vi "Main.vi"() -> ()   [LabVIEW 2020]
uses:
  <vilib>/Utility/error.llb/DialogType.ctl
  TypeDefs/SN_Enum.ctl
  <vilib>/numeric/Random Number (Range) DBL.vi
  <vilib>/ErrorRing/Error Ring.xnode
  <vilib>/Utility/SystemLogging/NI_SystemLogging.lvlib
panel:
  out "notification 2":bool
  out "notification 4":bool
  out "notification 1":bool
  out "notification 3":bool
  in  "Start Button":bool
  in  "View Button":bool
  out "error out":errorcluster
  in  "Abort Button":bool
  out "Tab Control":enum32{"Page 0", "Page 1", "Page 2"}(tab)
  in  "Save Button":bool
  in  "Path Control":path
  out "Grafica de Control":dbl(graph) caption="Waveform Chart - Dark"
  out "Torque Read":dbl
  in  "Torque Write":dbl
  out "Torque Read 2":dbl
  in  "Torque Write 2":dbl
  out "Torque Read 3":dbl
  in  "Tabs Buttons":enum32{"Button 1", "Button 2", "Button 3"}(radio)
  out "First Call: T/F":bool
  # "Debbugging Additional Objects"
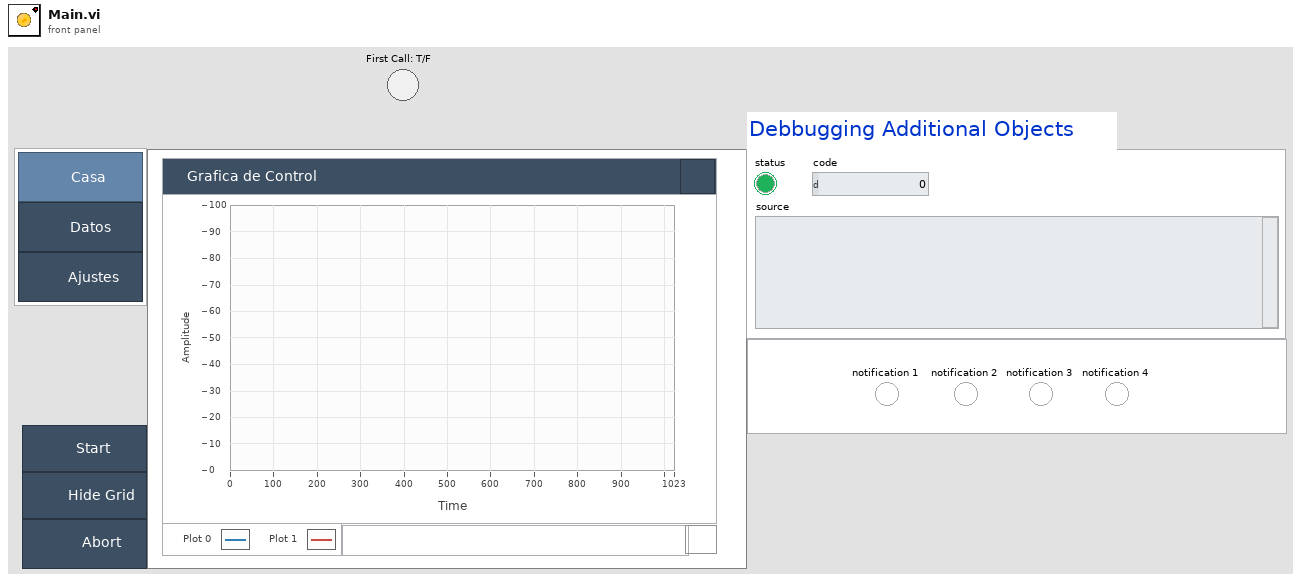
[diagram p1: front panel]
types:
  T1 = typedef "SN_Enum.ctl" = enum16{"Starting up", "Adquisition", "Save", "Fault"}
  T2 = typedef "DialogType.ctl" = u16
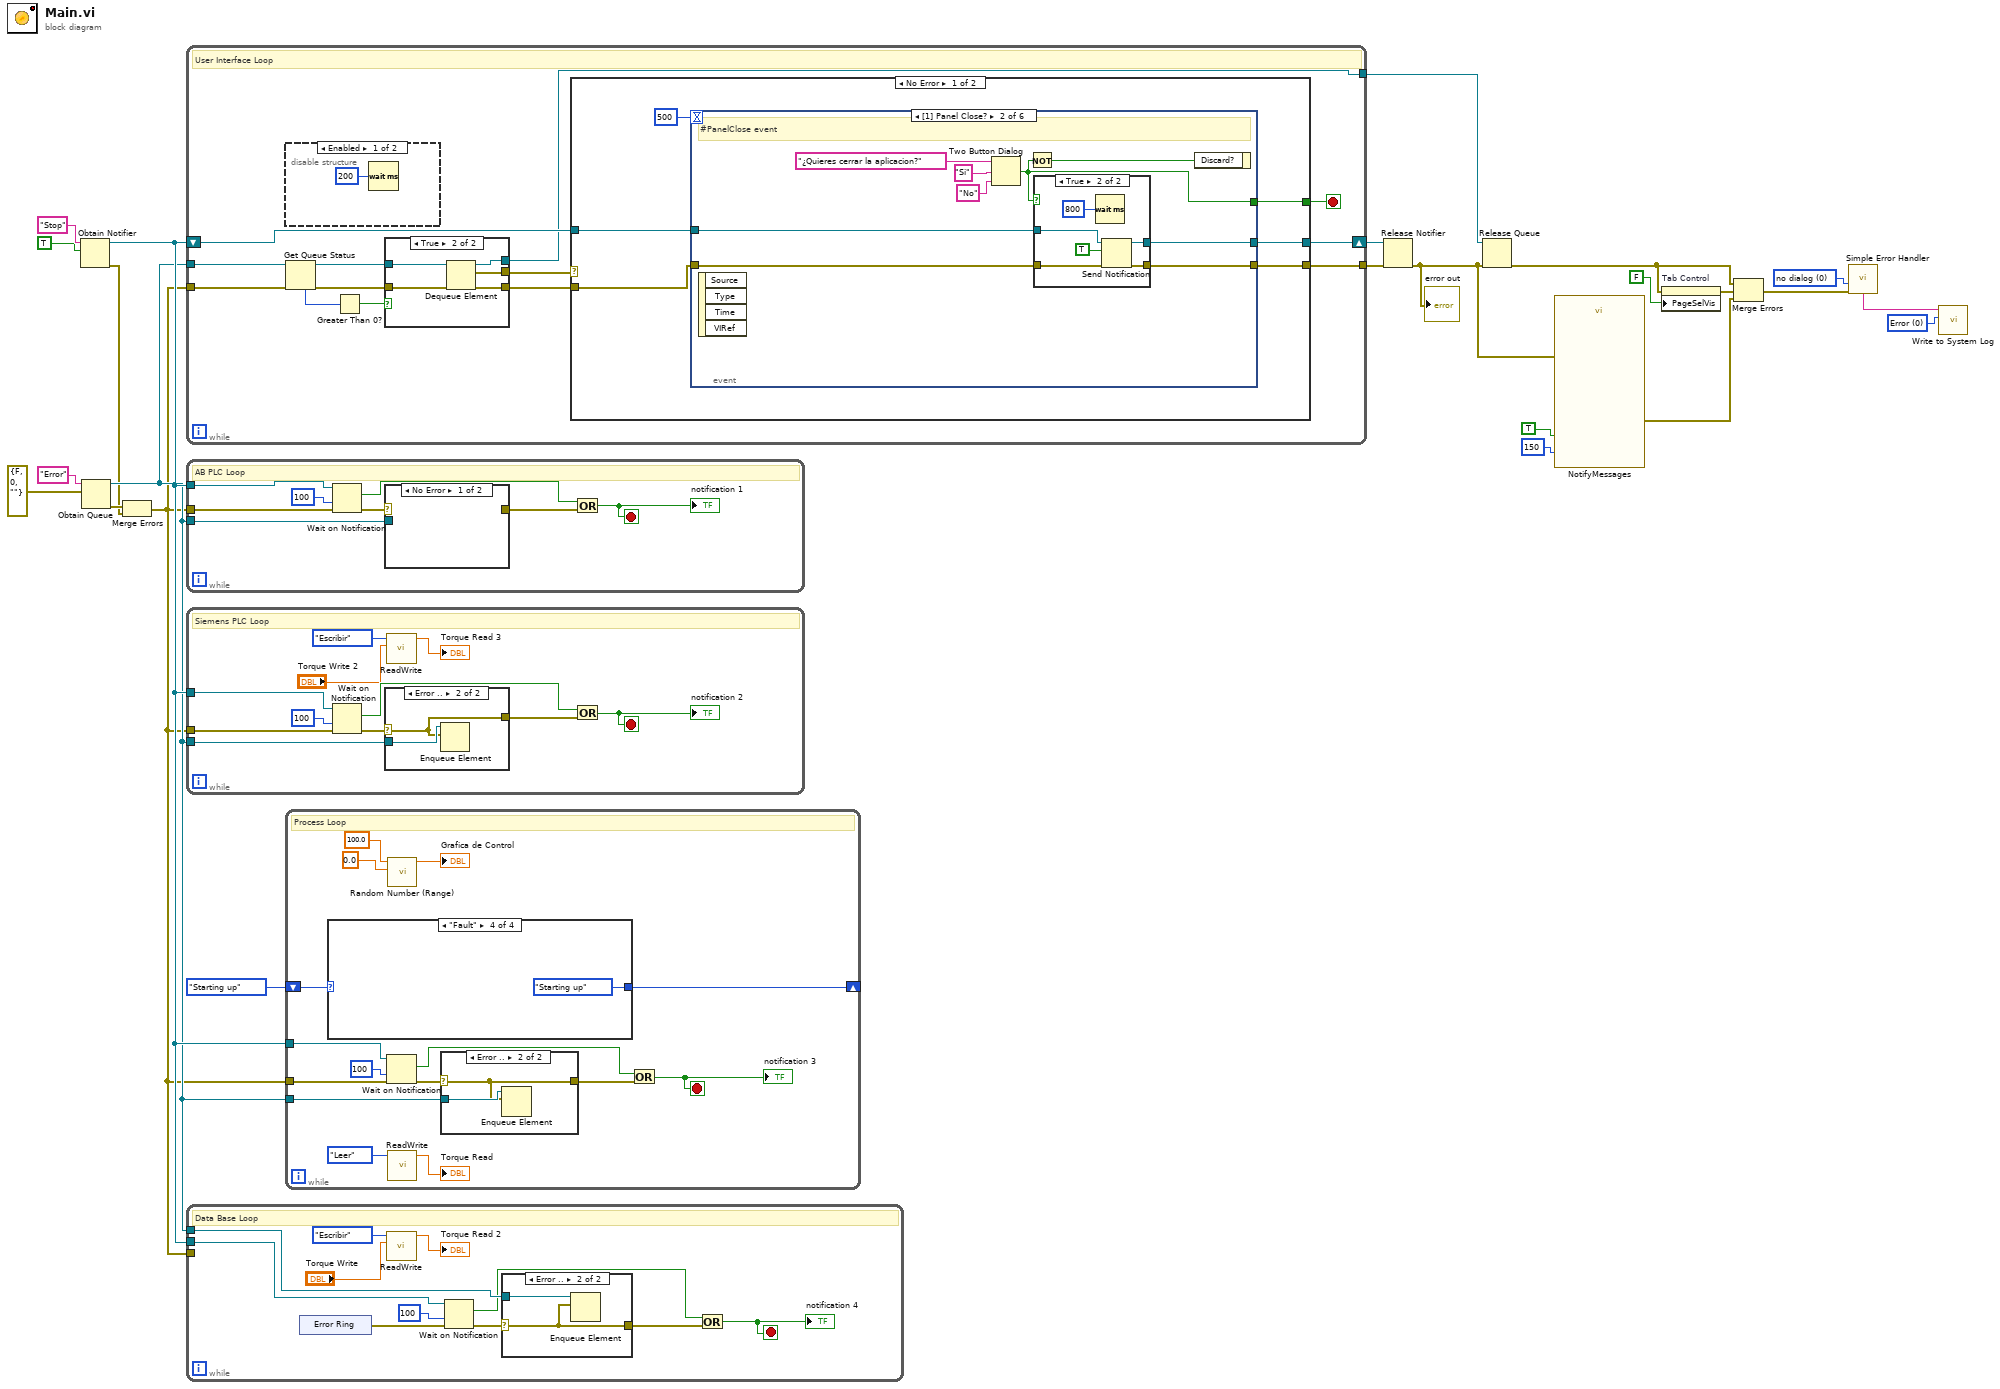
[diagram p0: block diagram]
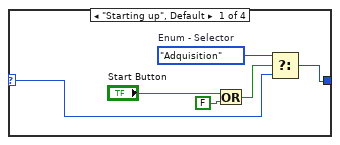
[diagram p3: hidden frame]
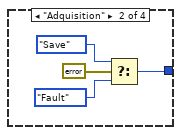
[diagram p4: hidden frame]
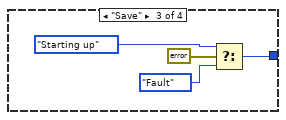
[diagram p5: hidden frame]
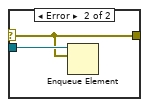
[diagram p8: hidden frame]
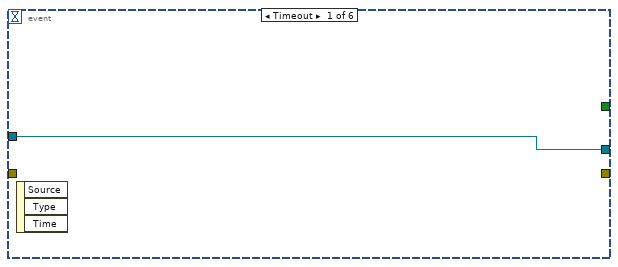
[diagram p9: hidden frame]
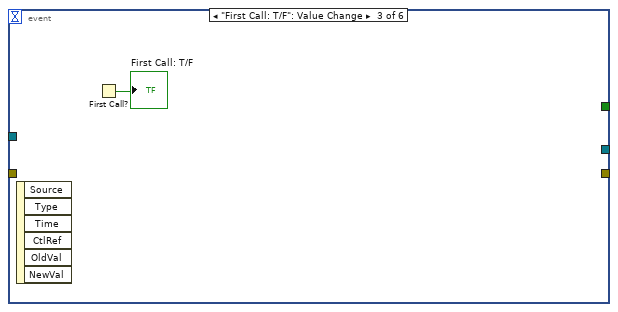
[diagram p11: hidden frame]
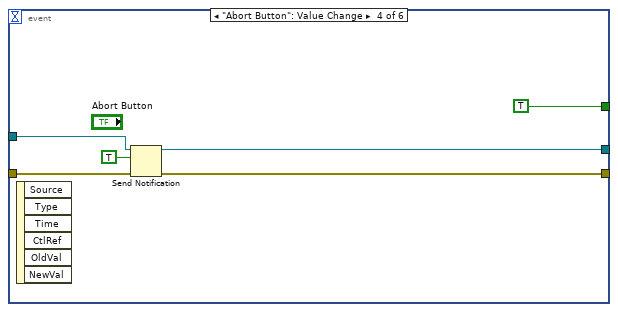
[diagram p12: hidden frame]
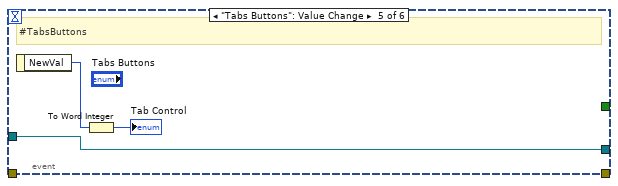
[diagram p13: hidden frame]
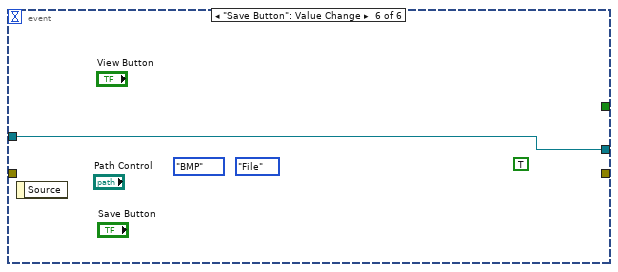
[diagram p14: hidden frame]
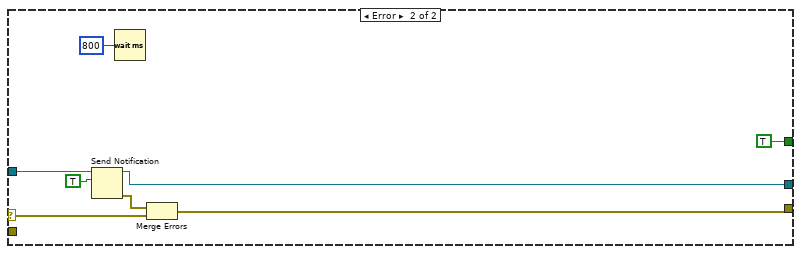
[diagram p15: hidden frame]
diagram:
  w11 = 0 items=["Error", "Warning", "Informational"] ("severity")
  w13 = T2 0 items=["no dialog", "OK message", "continue or stop message", "OK message + warnings", "continue/stop + warnings"] ("type of dialog (OK msg:1)")
  n1 = Obtain Notifier(name (unnamed)="Stop", notification data type=TRUE ("create if not found? (T)")) -> (notifier out=w22:refnum<notifier>, error out=w16:errorcluster)  [unwired: 2 in, 1 out]
  n2 = Obtain Queue(name (unnamed)="Error", element data type=errorcluster {FALSE, 0, ""}) -> (queue out=w19:refnum<queue>, error out=w17:errorcluster)  [unwired: 3 in, 1 out]
  n3 = Merge Errors(w17, w16) -> (w15:errorcluster)
  n4 = while {
    shift-right: [w35] -> w18
    shift-left: w22 -> [w36]
    tunnel: w19 -> [w34]
    tunnel: w15 -> [w29]
    tunnel: [w31] -> w14
    tunnel: [w25] -> w7
    stop <- w37 stop-if-true
    # "User Interface Loop"
    n5 = disable-structure shown="Enabled" {
      frame Enabled {
        n6 = Wait (ms)(milliseconds to wait=u32 200) -> ()  [unwired: 1 out]
      }
      frame Disabled {
      }
    }
    n7 = Get Queue Status(queue=w34, error in (no error)=w29) -> (queue out=w26:refnum<queue>, error out=w30:errorcluster, # elements in queue=w32:i32)  [unwired: 1 in, 5 out]
    n8 = Greater Than 0?(x=w32) -> (x > 0?=w33:bool)
    n9 = case shown="True" w33 {
      tunnel: w26 -> [w80 w85]
      tunnel: [_ w84] -> w27
      tunnel: w30 -> [_ w83]
      tunnel: [_ w82] -> w28
      tunnel: [w80 w81] -> w25
      frame False {
      }
      frame True {
        n10 = Dequeue Element(queue=w85, error in (no error)=w83) -> (queue out=w81:refnum<queue>, element=w82:errorcluster, error out=w84:errorcluster)  [unwired: 1 in, 1 out]
      }
    }
    n11 = case shown="No Error" w28 {
      selector: w28 -> [_ w72]
      tunnel: [w43 TRUE ("Abort Button")] -> w37
      tunnel: w36 -> [w41 w78]
      tunnel: [w40 w76] -> w35
      tunnel: w27 -> [w39 _]
      tunnel: [w38 w74] -> w31
      frame No Error {
        n12 = event shown="[1] Panel Close?" {
          selector: _ -> [_ _ _ _ _ _]
          dyn-events: _ -> [_ _ _ _ _ _]
          timeout: 500 -> [_ _ _ _ _ _]
          tunnel: [_ w49 _ TRUE ("Abort Button") _ _] -> w43
          tunnel: w41 -> [w44 w48 _ w66 w68 w71]
          tunnel: [w44 w47 _ w63 w68 w71] -> w40
          tunnel: w39 -> [_ w46 _ w64 _ _]
          tunnel: [_ w45 _ w62 _ _] -> w38
          event Timeout {
            n13 = event-data() -> ()  [unwired: 1 in, 3 out]
          }
          event Panel Close? {
            # "#PanelClose event"
            n14 = event-data() -> ()  [unwired: 1 in, 4 out]
            n15 = Two Button Dialog(message="¿Quieres cerrar la aplicacion?", 1:"No" ("F button name (\"Cancel\")"), 2:"Si" ("T button name (\"OK\")")) -> (T button?=w49:bool)
            n16 = Not(x=w49) -> (.not. x?=w50:bool)
            n17 = case shown="True" w49 {
              tunnel: w48 -> [w54 w59]
              tunnel: [w54 w58] -> w47
              tunnel: w46 -> [_ w56]
              tunnel: [_ w55] -> w45
              frame False {
              }
              frame True {
                n18 = Wait (ms)(milliseconds to wait=u32 800) -> ()  [unwired: 1 out]
                n19 = Send Notification(notification=TRUE, notifier=w59, error in (no error)=w56) -> (notifier out=w58:refnum<notifier>, error out=w55:errorcluster)
              }
            }
            n20 = event-data("Discard?"=w50) -> ()  [unwired: 1 in, 1 out]
          }
          event "First Call: T/F": Value Change {
            n21 = event-data() -> ()  [unwired: 1 in, 6 out]
            n22 = First Call?() -> (First Call?: T/F=→"First Call: T/F":bool)
          }
          event "Abort Button": Value Change {
            n23 = event-data() -> ()  [unwired: 1 in, 6 out]
            n24 = Send Notification(notification=TRUE, notifier=w66, error in (no error)=w64) -> (notifier out=w63:refnum<notifier>, error out=w62:errorcluster)
          }
          event "Tabs Buttons": Value Change {
            # "#TabsButtons"
            n25 = event-data() -> ("NewVal"=w70:enum32{"Button 1", "Button 2", "Button 3"})  [unwired: 1 in]
            n26 = To Word Integer(number=w70) -> (16bit integer=→"Tab Control":i16)
          }
          event "Save Button": Value Change {
            (unwired) TRUE ("Always Overwrite")
            (unwired) enum32{"File", "Clipboard"}."File" ("Target")
            (unwired) enum32{"BMP", "EPS", "EMF", "PICT"}."BMP" ("File Type")
            n27 = event-data() -> ()  [unwired: 1 in, 1 out]
          }
        }
      }
      frame Error {
        n28 = Send Notification(notification=TRUE, notifier=w78) -> (notifier out=w76:refnum<notifier>, error out=w73:errorcluster)  [unwired: 1 in]
        n29 = Wait (ms)(milliseconds to wait=u32 800) -> ()  [unwired: 1 out]
        n30 = Merge Errors(w73, w72) -> (w74:errorcluster)
      }
    }
  }
  n31 = while {
    tunnel: w22 -> [w93]
    tunnel: w15 -> [w92]
    tunnel: w19 -> [w91]
    stop <- w87 stop-if-true
    # "AB PLC Loop"
    n32 = Wait on Notification(notifier=w93, timeout in ms (-1)=100, error in (no error)=w92) -> (notification=w90:bool, error out=w89:errorcluster)  [unwired: 1 in, 2 out]
    n33 = case shown="No Error" w89 {
      selector: w89 -> [_ w95]
      tunnel: w91 -> [_ w96]
      tunnel: [_ w95] -> w88
      frame No Error {
      }
      frame Error {
        n34 = Enqueue Element(queue=w96, element=w95) -> ()  [unwired: 2 in, 3 out]
      }
    }
    n35 = Or(x=w90, y=w88) -> (x .or. y?=w87:bool)
    "notification 1" <- w87
  }
  n36 = while {
    tunnel: w22 -> [w106]
    tunnel: w15 -> [w105]
    tunnel: w19 -> [w104]
    stop <- w100 stop-if-true
    # "Siemens PLC Loop"
    n37 = Wait on Notification(notifier=w106, timeout in ms (-1)=100, error in (no error)=w105) -> (notification=w103:bool, error out=w101:errorcluster)  [unwired: 1 in, 2 out]
    n38 = case shown="Error .." w101 {
      selector: w101 -> [_ w108]
      tunnel: w104 -> [_ w109]
      tunnel: [_ w108] -> w102
      frame No Error {
      }
      frame Error {
        n39 = Enqueue Element(queue=w109, element=w108) -> ()  [unwired: 2 in, 3 out]
      }
    }
    n40 = call "ReadWrite.vi"("Torque Write"="Torque Write 2", "Selector FGV"=enum16{"Leer", "Escribir"}."Escribir") -> ("Torque Read"=→"Torque Read 3":dbl)  [unwired: 9 in]
    n41 = Or(x=w103, y=w102) -> (x .or. y?=w100:bool)
    "notification 2" <- w100
  }
  n42 = while {
    tunnel: w22 -> [w119]
    tunnel: w19 -> [w118]
    tunnel: w15 -> [_]
    stop <- w110 stop-if-true
    # "Data Base Loop"
    n43 = xnode "Error Ring"() -> ("error out"=w114:errorcluster)
    n44 = call "ReadWrite.vi"("Torque Write"="Torque Write", "Selector FGV"=enum16{"Leer", "Escribir"}."Escribir") -> ("Torque Read"=→"Torque Read 2":dbl)  [unwired: 9 in]
    n45 = Wait on Notification(notifier=w119, timeout in ms (-1)=100, error in (no error)=w114) -> (notification=w117:bool, error out=w116:errorcluster)  [unwired: 1 in, 2 out]
    n46 = case shown="Error .." w116 {
      selector: w116 -> [_ w122]
      tunnel: w118 -> [_ w123]
      tunnel: [_ w122] -> w115
      frame No Error {
      }
      frame Error {
        n47 = Enqueue Element(queue=w123, element=w122) -> ()  [unwired: 2 in, 3 out]
      }
    }
    n48 = Or(x=w117, y=w115) -> (x .or. y?=w110:bool)
    "notification 4" <- w110
  }
  n49 = while {
    tunnel: w22 -> [w137]
    tunnel: w15 -> [w136]
    tunnel: w19 -> [w135]
    shift-right: [w128] -> _
    shift-left: SN_Enum."Starting up" ("Enum - Selector") -> [w129]
    stop <- w124 stop-if-true
    # "Process Loop"
    n50 = case shown="\"Fault\"" w129 {
      selector: w129 -> [w139 _ _ _]
      tunnel: [w140 w148 w152 SN_Enum."Starting up" ("Enum - Selector")] -> w128
      frame "Starting up", Default {
        w142 = SN_Enum."Adquisition"  # Enum - Selector
        n51 = Or(x="Start Button", y=FALSE) -> (x .or. y?=w143:bool)
        n52 = Select(t=w142, s=w143, f=w139) -> (s? t:f=w140:T1)
      }
      frame "Adquisition" {
        n53 = Select(t=SN_Enum."Save" ("Enum - Selector"), s=errorcluster {"status"=FALSE, "code"=0, "source"=""} ("error constant"), f=SN_Enum."Fault" ("Enum - Selector")) -> (s? t:f=w148:T1)
      }
      frame "Save" {
        n54 = Select(t=SN_Enum."Starting up" ("Enum - Selector"), s=errorcluster {"status"=FALSE, "code"=0, "source"=""} ("error constant"), f=SN_Enum."Fault" ("Enum - Selector")) -> (s? t:f=w152:T1)
      }
      frame "Fault" {
      }
    }
    n55 = Wait on Notification(notifier=w137, timeout in ms (-1)=100, error in (no error)=w136) -> (notification=w134:bool, error out=w133:errorcluster)  [unwired: 1 in, 2 out]
    n56 = call-poly <vilib>:"Random Number (Range).vi"("lower bound (0)"=0.0, "upper bound (100)"=100.0) -> ("number"=→"Grafica de Control":dbl)  [unwired: 9 in]
    n57 = call "ReadWrite.vi"("Selector FGV"=enum16{"Leer", "Escribir"}."Leer") -> ("Torque Read"=→"Torque Read":dbl)  [unwired: 10 in]
    n58 = case shown="Error .." w133 {
      selector: w133 -> [_ w154]
      tunnel: w135 -> [_ w155]
      tunnel: [_ w154] -> w132
      frame No Error {
      }
      frame Error {
        n59 = Enqueue Element(queue=w155, element=w154) -> ()  [unwired: 2 in, 3 out]
      }
    }
    n60 = Or(x=w134, y=w132) -> (x .or. y?=w124:bool)
    "notification 3" <- w124
  }
  n61 = Release Notifier(notifier=w18, error in (no error)=w14) -> (error out=w5:errorcluster)  [unwired: 1 in, 2 out]
  "error out" <- w5
  n62 = Release Queue(queue=w7, error in (no error)=w5) -> (error out=w6:errorcluster)  [unwired: 1 in, 2 out]
  n63 = call "NotifyMessages.vi"("Add Alarm Button"=TRUE, "milliseconds to wait"=u32 150, "error in (no error)"=w5) -> ("error out"=w4:errorcluster)  [unwired: 8 in]
  n64 = property on="Tab Control" class="TabCtl (strict)"(error in=w6, "PageSelVis"=FALSE ("Page Selector Visible")) -> (error out=w9:errorcluster)  [unwired: 1 in, 1 out]
  n65 = Merge Errors(w6, w9, w4) -> (w8:errorcluster)
  n66 = call <vilib>:"Simple Error Handler.vi"("type of dialog (OK msg:1)"=w13, "error in (no error)"=w8) -> ("message"=w12:string)  [unwired: 3 in, 4 out]
  n67 = call <vilib>:"Write to System Log.vi"("severity"=w11, "message"=w12) -> ()  [unwired: 9 in, 1 out]
